vi "Agilent VNA Convert Form 2 Data.vi"(8 "Raw Data Point":string) -> (0 "Number":cdb)   [LabVIEW 2011]
panel:
  out "Single Array":sgl[](array[numeric])
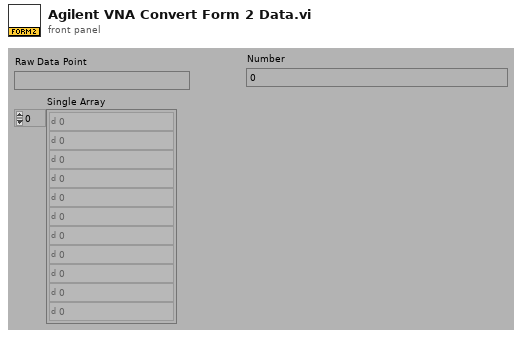
[diagram p1: front panel]
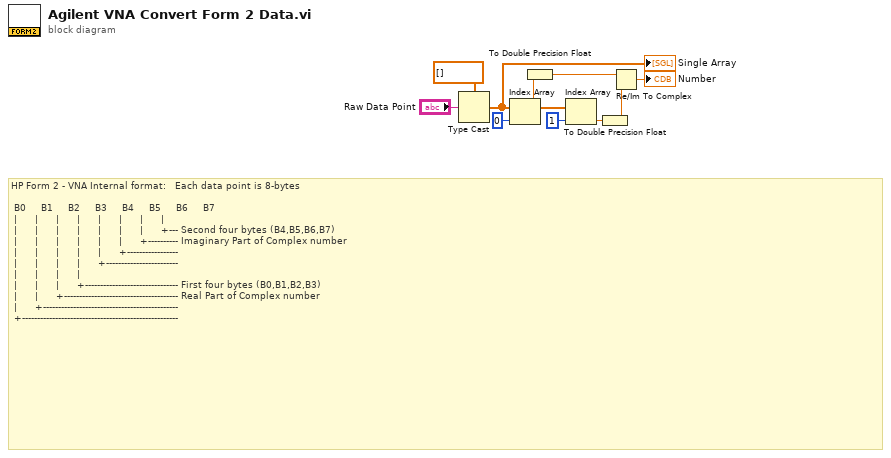
[diagram p0: block diagram]
diagram:
  # "HP Form 2 - VNA Internal format:   Each data point is 8-bytes\n\n B0     B1     B2     B3     B4     B5     B6     B7\n |      |      |      |      |      |      |      |\n |      |      |      |      |      |      |      +--- Second four bytes (B4,B5,B6,B7)\n |      |      |      |      |      |      +---------- Imaginary Part of Complex number\n |      |      |      |      |      +-----------------\n |      |      |      |      +------------------------\n |      |      |      |\n |      |      |      +------------------------------- First four bytes (B0,B1,B2,B3)\n |      |      +-------------------------------------- Real Part of Complex number\n |      +---------------------------------------------\n +----------------------------------------------------"
  n1 = Type Cast(type=sgl[] [], x="Raw Data Point") -> (*(type *) &x=w2:sgl[])
  "Single Array" <- w2
  n2 = Index Array(array=w2, index=0) -> (element=w5:sgl)
  n3 = To Double Precision Float(number=w5) -> (double precision float=w4:dbl)
  n4 = Index Array(array=w2, index=1) -> (element=w7:sgl)
  n5 = To Double Precision Float(number=w7) -> (double precision float=w6:dbl)
  n6 = Re/Im To Complex(1:w6, 2:w4) -> (0:→"Number":cdb)
